vi "Panel.vi"(11 "ImageButtonEditorPanel in":refnum<class "ImageButtonEditorPanel.lvclass">) -> ()   [LabVIEW 2020, in "VolatusGUIControls.lvlib" / "ImageButtonEditorPanel.lvclass"]
uses:
  ImageButtonEditorPanel.lvclass
  C:/dev/lv20CE/relink/volatus-gui-controls/VolatusGUIEditorCore/ElementEditorPanel/ElementEditorPanel.lvclass
  C:/dev/lv20CE/relink/lv-oopanel/OOPanel/Panel/Panel.lvclass
  lv-oopanel/OOPanel/Panel/Basic UI State.ctl
  lv-autocomplete/AutoComplete/AutoComplete/AutoComplete.lvclass/AutoComplete.ctl
  ImageButtonEditorPanel.lvclass/ImageButtonEditorPanel.ctl
  lv-autocomplete/AutoComplete/Launch Autocomplete Handler.vi
  lv-autocomplete/AutoComplete/AutoComplete/AutoComplete.lvclass
  lv-oopanel/OOPanel/Panel/Panel.lvclass
  lv-oopanel/OOPanel/OOPanel.lvlib
  VolatusGUIEditorCore/ElementEditorPanel/ElementEditorPanel.lvclass
  VolatusGUIEditorCore/VolatusGUIEditorCore.lvlib
  lv-web-crypto/lv-base64/Base64.lvlib
  C:/dev/lv20CE/relink/volatus-gui-controls/VolatusGUIControls/ImageButtonEditorPanel/ImageButtonEditorPanel.lvclass
panel:
  out "Last True Image":string
  out "Last False Image":string
  out "Last Image Folder":path
  in  "Top":i32
  in  "Left":i32
  in  "Select True":bool
  in  "Select False":bool
  out "True":picture
  out "False":picture
  in  "Label Text Color":u32(colorbox) caption="Color"
  in  "Label Visible":bool caption="Visible"
  in  "Label":string
  in  "Channel":string
  # "Label"
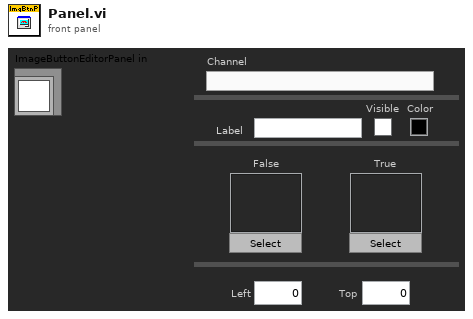
[diagram p1: front panel]
types:
  T1 = typedef "OOPanel.lvlib/Panel.lvclass/Basic UI State.ctl" = enum16{"Init", "Run", "Close"}
  T2 = typedef "VolatusGUIEditorCore.lvlib/ElementEditorPanel.lvclass/Incoming Events.ctl" = cluster{"Update Control":refnum<user-event>}
  T3 = typedef "OOPanel.lvlib/Panel.lvclass/Panel Events.ctl" = cluster{"Visbility":refnum<user-event>, "Close":refnum<user-event>}
  T4 = typedef "VolatusGUIControls.lvlib/ImageButtonEditorPanel.lvclass/Props.ctl" = cluster{"JSON":T5, "Label":T6, "Position":T7}
  T5 = typedef "VolatusGUIControls.lvlib/ImageButtonEditorPanel.lvclass/JSON Props.ctl" = cluster{"Channel":string, "FalseImage":string, "TrueImage":string}
  T6 = typedef "VolatusGUIEditorCore.lvlib/Label Props.ctl" = cluster{"Text":string, "Text Color":u32, "Visible":bool}
  T7 = typedef "VolatusGUIEditorCore.lvlib/Position Props.ctl" = cluster{"Left":i32, "Top":i32}
  T8 = typedef "OOPanel.lvlib/Visibility State.ctl" = enum16{"Idle", "Closed", "Hidden", "Visible", "Subpanel", "Hidden Subpanel"}
  T9 = cluster{"Label":string, "Label Text Color":u32, "Label Visible":bool}
  T10 = typedef "imagedata.ctl" = cluster{"image type":i32, "image depth":i32, "image":u8[], "mask":u8[], "colors":u32[], "Rectangle":cluster{"left":i16, "top":i16, "right":i16, "bottom":i16}}
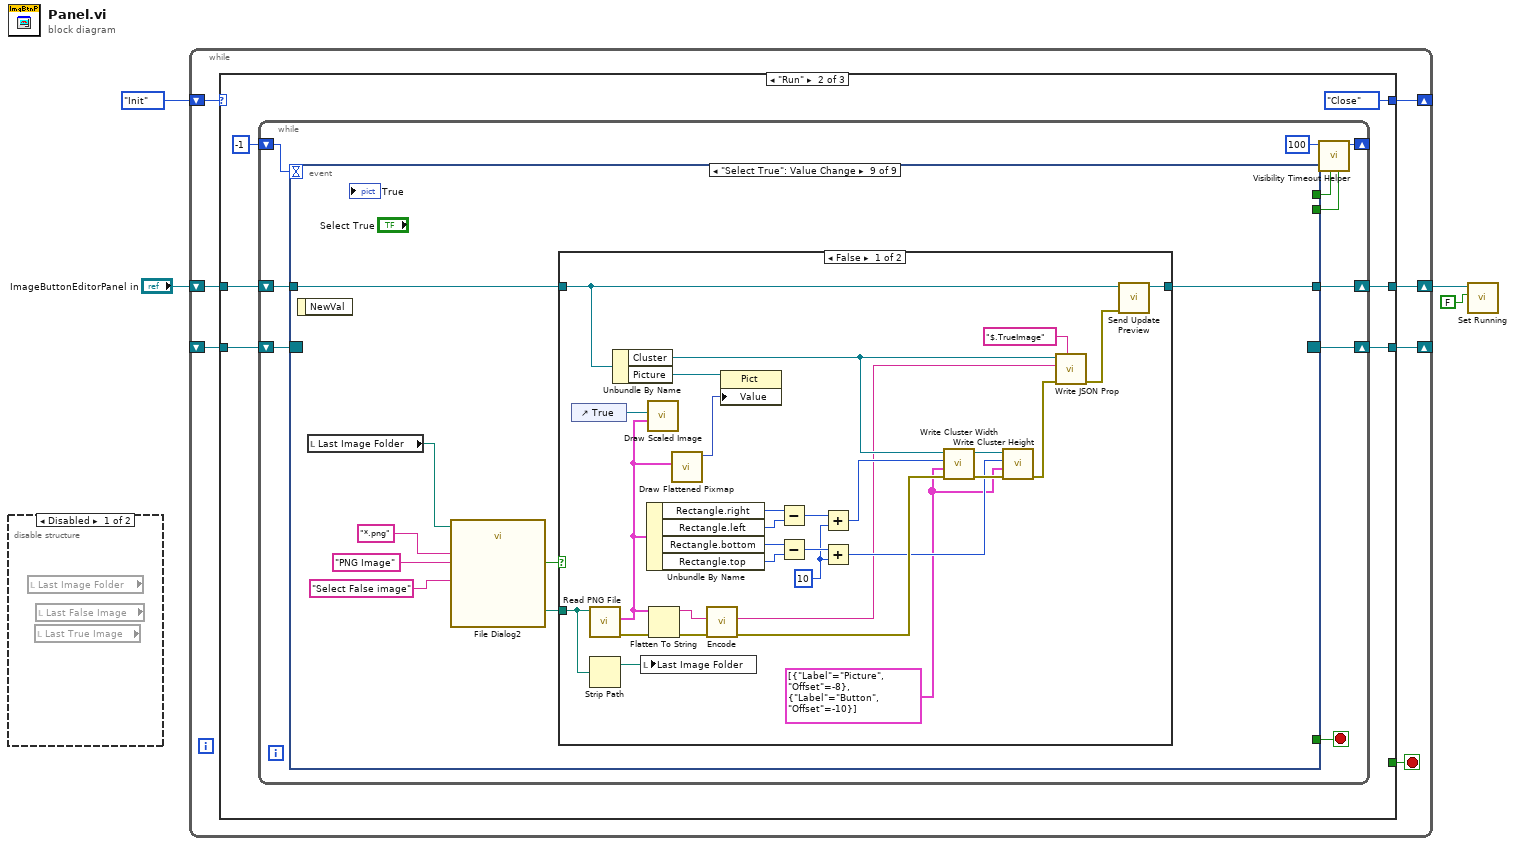
[diagram p0: block diagram]
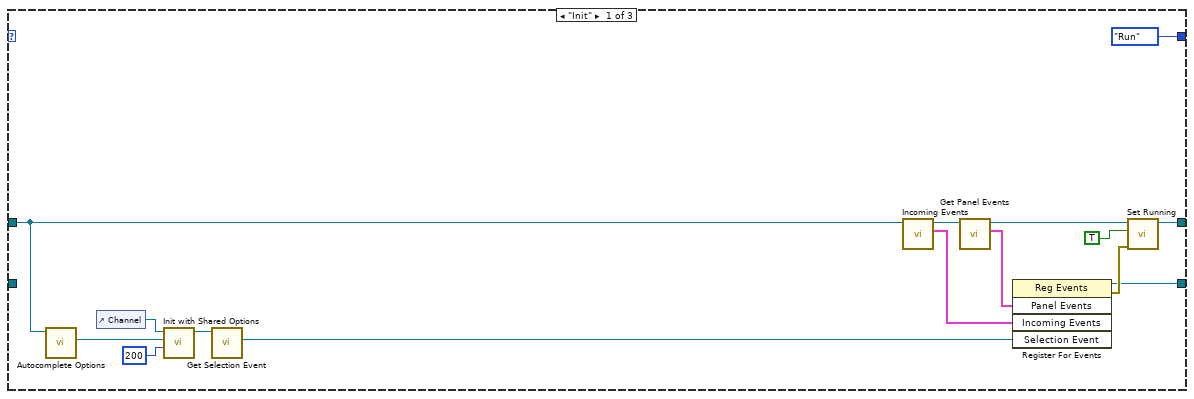
[diagram p3: hidden frame]
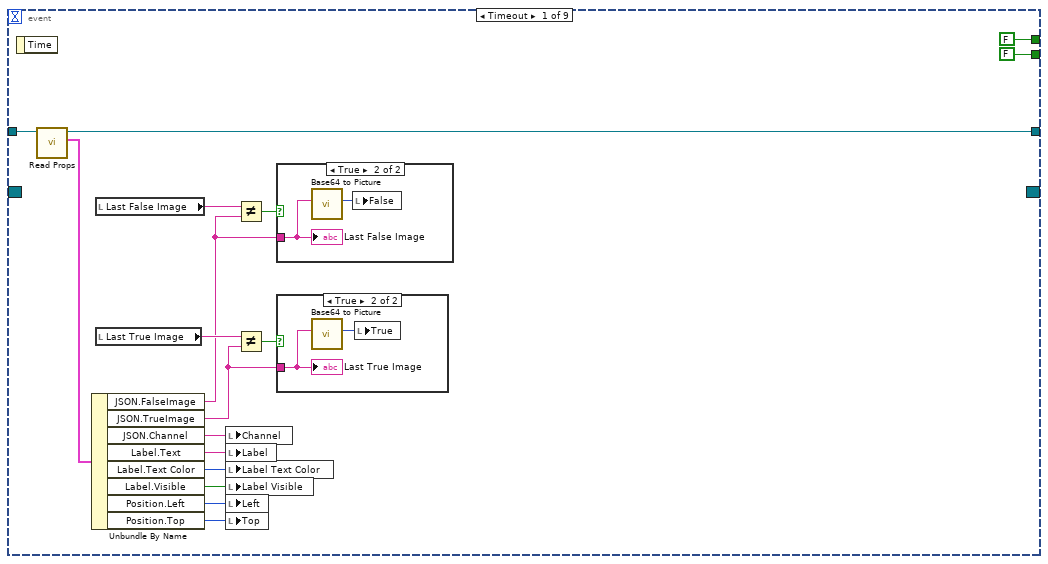
[diagram p4: hidden frame]
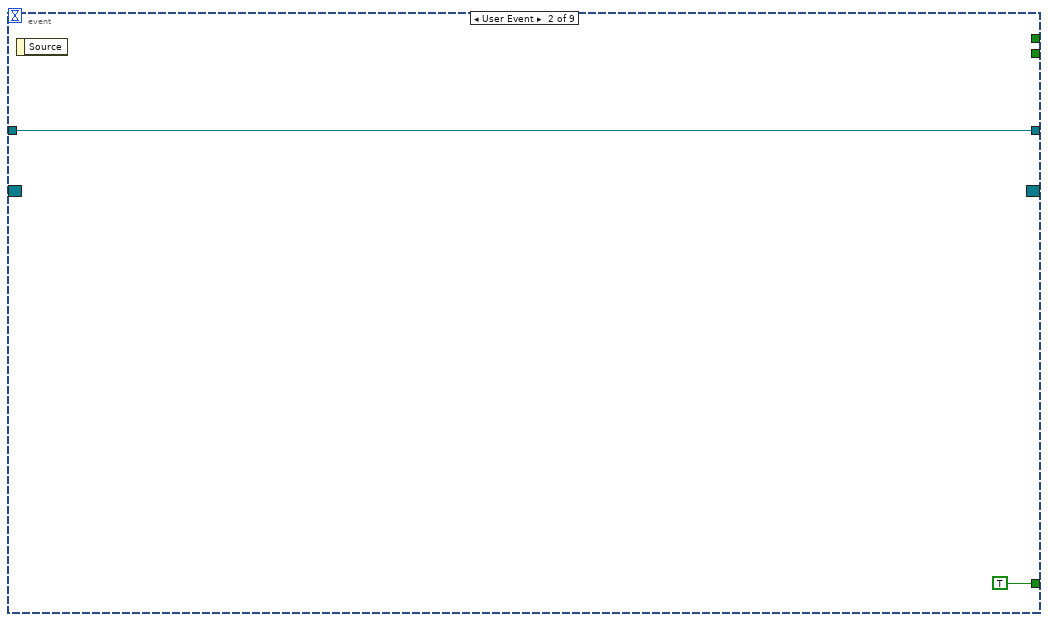
[diagram p7: hidden frame]
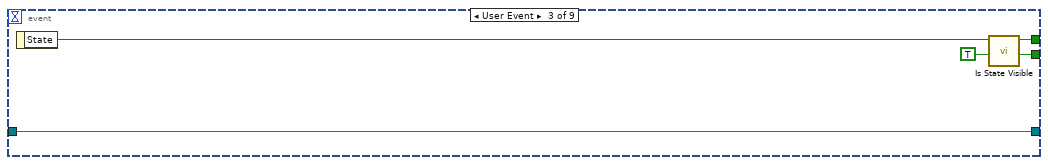
[diagram p8: hidden frame]
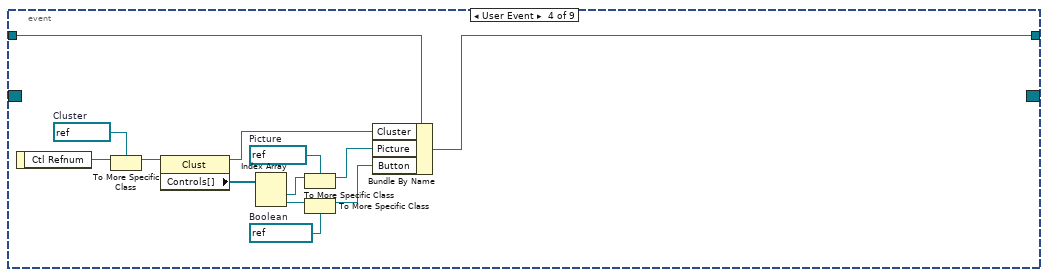
[diagram p9: hidden frame]
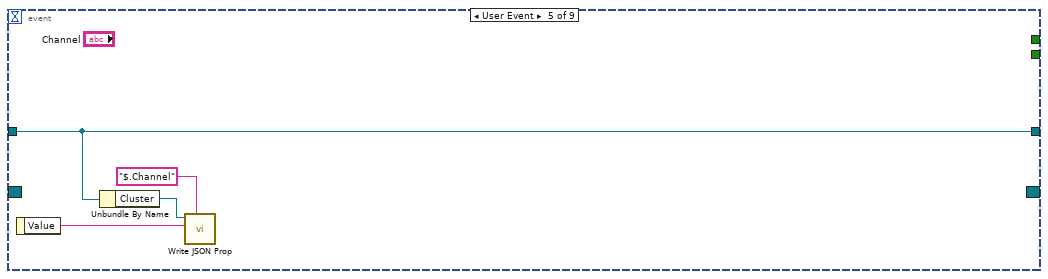
[diagram p10: hidden frame]
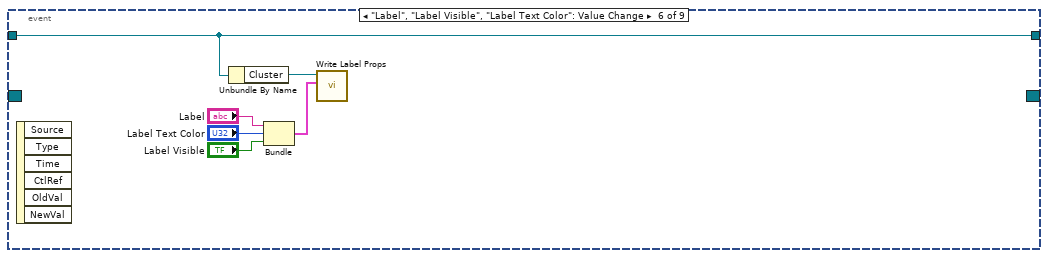
[diagram p11: hidden frame]
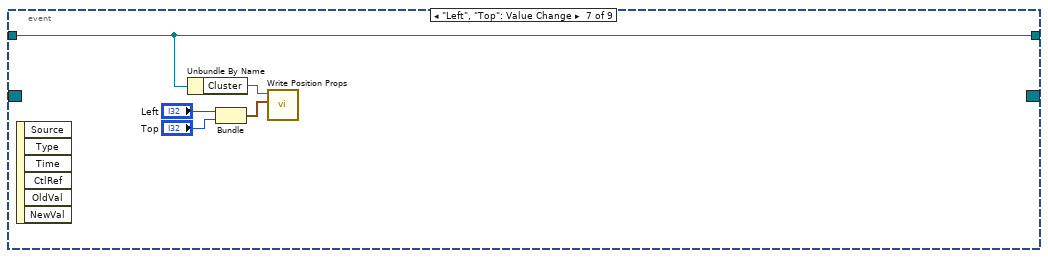
[diagram p12: hidden frame]
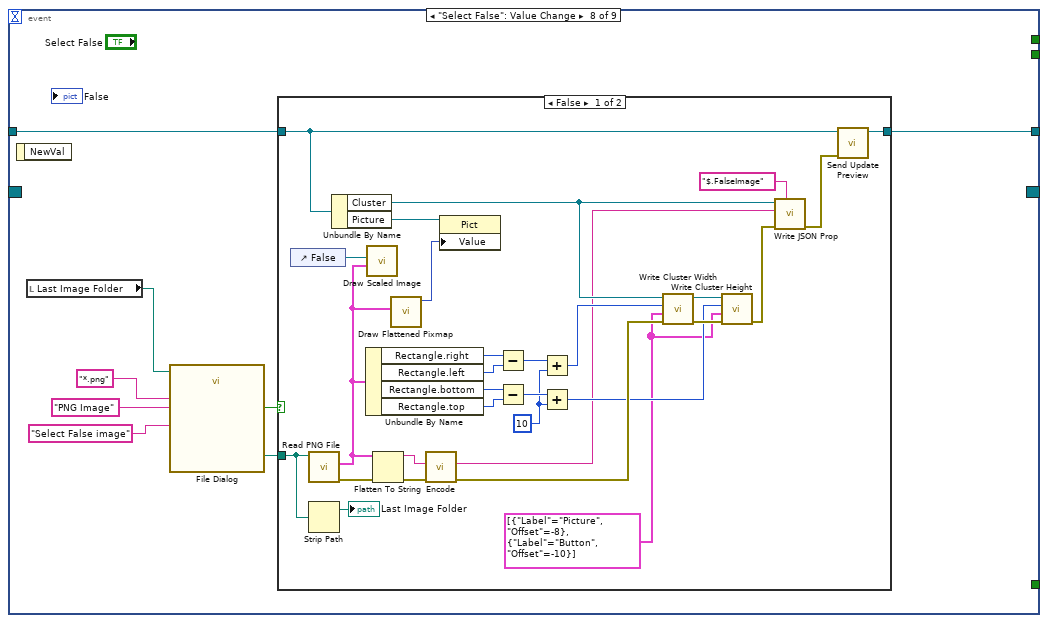
[diagram p13: hidden frame]
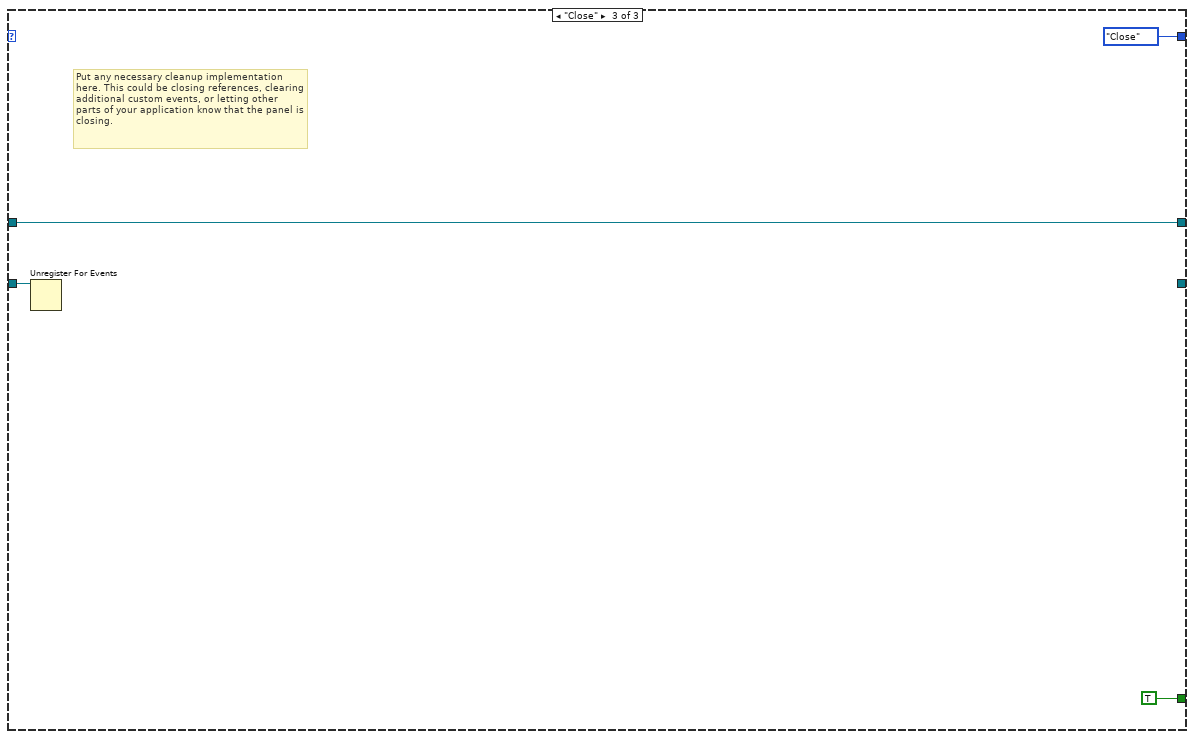
[diagram p16: hidden frame]
diagram:
  n1 = disable-structure shown="Disabled" {
    frame Disabled {
      n2 = local read "Last Image Folder"() -> ()  [unwired: 1 out]
      n3 = local read "Last True Image"() -> ()  [unwired: 1 out]
      n4 = local read "Last False Image"() -> ()  [unwired: 1 out]
    }
    frame Enabled {
    }
  }
  n5 = while {
    shift-right: [w10] -> _
    shift-left: _ -> [w11]
    shift-right: [w8] -> _
    shift-left: Basic_UI_State."Init" ("Basic UI State") -> [w9]
    shift-right: [w6] -> w4
    shift-left: "ImageButtonEditorPanel in" -> [w5]
    stop <- w7 stop-if-true
    n6 = case shown="\"Run\"" w9 {
      tunnel: w11 -> [_ w32 w175]
      tunnel: [w23 w30 _] -> w10
      tunnel: [Basic_UI_State."Run" ("Basic UI State") Basic_UI_State."Close" ("Basic UI State") Basic_UI_State."Close" ("Basic UI State")] -> w8
      tunnel: [_ _ TRUE] -> w7
      tunnel: [w22 w27 w174] -> w6
      tunnel: w5 -> [w14 w28 w174]
      frame "Init" {
        n7 = call "Autocomplete Options.vi"("ElementEditorPanel in"=w14) -> ("Autocomplete Options"=w17:refnum<class "Shared Options.lvclass">)  [unwired: 10 in]
        n8 = control-ref of="Channel"() -> (w13:refnum<vi>)
        n9 = call "Init with Shared Options.vi"("Height (200)"=i16 200, "Shared Options"=w17, "Str Refnum"=w13) -> ("AutoComplete out"=w16:refnum<class "AutoComplete.lvclass">)  [unwired: 7 in, 1 out]
        n10 = call "Get Selection Event.vi"("AutoComplete in"=w16) -> ("Selection Event"=w12:refnum<user-event>)  [unwired: 9 in, 1 out]
        n11 = call "Incoming Events.vi"("ElementEditorPanel in"=w14) -> ("Incoming Events"=w18:T2, "ElementEditorPanel out"=w19:refnum<class "ImageButtonEditorPanel.lvclass">)  [unwired: 9 in]
        n12 = call "Get Panel Events.vi"("Panel in"=w19) -> ("Panel Events"=w20:T3, "Panel out"=w21:refnum<class "ImageButtonEditorPanel.lvclass">)  [unwired: 8 in, 1 out]
        n13 = register-events(w20, w18, w12) -> (reference out=w23:refnum<event-registration>, error out=w25:errorcluster)  [unwired: 2 in]
        n14 = call "Set Running.vi"("error in (no error)"=w25, "Running"=TRUE, "Panel in"=w21) -> ("Panel out"=w22:refnum<class "ImageButtonEditorPanel.lvclass">)  [unwired: 7 in, 1 out]
      }
      frame "Run" {
        n15 = while {
          shift-right: [w38] -> w30
          shift-left: w32 -> [w39]
          shift-right: [w41] -> _
          shift-left: -1 ("Timeout") -> [w40]
          shift-right: [w33] -> w27
          shift-left: w28 -> [w34]
          stop <- w35 stop-if-true
          n16 = event shown="[8] \"Select True\": Value Change" {
            selector: w39 -> [_ _ _ _ _ _ _ _ _]
            dyn-events: [_ _ _ _ _ _ _ _ _] -> w38
            timeout: w40 -> [_ _ _ _ _ _ _ _ _]
            tunnel: [FALSE _ w68 _ _ _ _ _ _] -> w37
            tunnel: [FALSE _ TRUE _ _ _ _ _ _] -> w36
            tunnel: [_ TRUE _ _ _ _ _ _ _] -> w35
            tunnel: w34 -> [w55 w64 w66 w82 w84 w88 w94 w100 w138]
            tunnel: [w56 w64 w66 w73 w84 w88 w94 w99 w137] -> w33
            event Timeout {
              n17 = event-data() -> ()  [unwired: 1 in, 1 out]
              n18 = call "Read Props.vi"("ImageButtonEditorPanel in"=w55) -> ("Props"=w57:T4, "ImageButtonEditorPanel out"=w56:refnum<class "ImageButtonEditorPanel.lvclass">)  [unwired: 8 in, 1 out]
              n19 = Unbundle By Name(w57) -> ("JSON.FalseImage"=w45:string, "JSON.TrueImage"=w43:string, "JSON.Channel"=w54:string, "Label.Text"=w52:string, "Label.Text Color"=w51:u32, "Label.Visible"=w50:bool, "Position.Left"=w49:i32, "Position.Top"=w53:i32)
              n20 = local read "Last False Image"() -> (w48:string)
              n21 = local read "Last True Image"() -> (w47:string)
              n22 = local write "Channel"(w54) -> ()
              n23 = local write "Label"(w52) -> ()
              n24 = local write "Label Text Color"(w51) -> ()
              n25 = local write "Label Visible"(w50) -> ()
              n26 = local write "Left"(w49) -> ()
              n27 = local write "Top"(w53) -> ()
              n28 = Not Equal?(x=w48, y=w45) -> (x != y?=w46:bool)
              n29 = Not Equal?(x=w47, y=w43) -> (x != y?=w44:bool)
              n30 = case shown="True" w46 {
                tunnel: w45 -> [_ w63]
                frame False {
                }
                frame True {
                  n31 = call "Base64 to Picture.vi"("Base64 PNG Data"=w63) -> ("Picture"=w62:picture)  [unwired: 9 in, 1 out]
                  n32 = local write "False"(w62) -> ()
                  "Last False Image" <- w63
                }
              }
              n33 = case shown="True" w44 {
                tunnel: w43 -> [_ w61]
                frame False {
                }
                frame True {
                  n34 = call "Base64 to Picture.vi"("Base64 PNG Data"=w61) -> ("Picture"=w60:picture)  [unwired: 9 in, 1 out]
                  n35 = local write "True"(w60) -> ()
                  "Last True Image" <- w61
                }
              }
            }
            event User Event {
              n36 = event-data() -> ()  [unwired: 1 in, 1 out]
            }
            event User Event {
              n37 = event-data() -> ("State"=w69:T8)  [unwired: 1 in]
              n38 = call "Is State Visible.vi"("Visibility"=w69) -> ("Visible"=w68:bool)  [unwired: 10 in]
            }
            event User Event {
              w75 = refnum<vi> refnum  # Boolean
              w77 = refnum<vi> refnum  # Picture
              w80 = refnum<vi> refnum  # Cluster
              n39 = event-data() -> ("Ctl Refnum"=w81:refnum<vi>)  [unwired: 1 in]
              n40 = To More Specific Class(target class=w80, reference=w81) -> (specific class reference=w79:refnum<vi>)  [unwired: 1 in, 1 out]
              n41 = property class="Clust"(reference=w79) -> (reference out=w72:refnum<vi>, "Controls[]"=w78:refnum<vi>[])  [unwired: 1 in, 1 out]
              n42 = Index Array(array=w78) -> (element #1=w76:refnum<vi>, element #2=w74:refnum<vi>)  [unwired: 2 in]
              n43 = To More Specific Class(target class=w77, reference=w76) -> (specific class reference=w71:refnum<vi>)  [unwired: 1 in, 1 out]
              n44 = To More Specific Class(target class=w75, reference=w74) -> (specific class reference=w70:refnum<vi>)  [unwired: 1 in, 1 out]
              n45 = Bundle By Name(cluster=w82, "Cluster"=w72, "Picture"=w71, "Button"=w70) -> (w73:refnum<class "ImageButtonEditorPanel.lvclass">)
            }
            event User Event {
              n46 = event-data() -> ("Value"=w83:string)  [unwired: 1 in]
              n47 = Unbundle By Name(w84) -> ("Cluster"=w86:refnum<vi>)
              n48 = call "Write JSON Prop.vi"("JSON Path"="$.Channel" ("$Path or Item Name"), "Value"=w83, "Ctl Refnum in"=w86) -> ()  [unwired: 7 in, 2 out]
            }
            event "Label", "Label Visible", "Label Text Color": Value Change {
              n49 = event-data() -> ()  [unwired: 1 in, 6 out]
              n50 = Unbundle By Name(w88) -> ("Cluster"=w87:refnum<vi>)
              n51 = Bundle("Label"="Label", "Label Text Color"="Label Text Color", "Label Visible"="Label Visible") -> (w89:T9)  [unwired: 1 in]
              n52 = call "Write Label Props.vi"("Label Props"=w89, "Ctl Refnum in"=w87) -> ()  [unwired: 8 in, 2 out]
            }
            event "Left", "Top": Value Change {
              n53 = event-data() -> ()  [unwired: 1 in, 6 out]
              n54 = Unbundle By Name(w94) -> ("Cluster"=w93:refnum<vi>)
              n55 = Bundle("Left"="Left", "Top"="Top") -> (w95:cluster{"Left":i32, "Top":i32})  [unwired: 1 in]
              n56 = call "Write Position Props.vi"("Position Props"=w95, "Ctl Refnum in"=w93) -> ()  [unwired: 8 in, 2 out]
            }
            event "Select False": Value Change {
              n57 = event-data() -> ()  [unwired: 1 in, 1 out]
              n58 = local read "Last Image Folder"() -> (w98:path)
              n59 = call "File Dialog"("start path"=w98, "prompt"="Select False image", "pattern (all files)"="*.png", "pattern label"="PNG Image") -> ("selected path"=w101:path, "cancelled"=w102:bool)  [unwired: 8 in, 2 out]
              n60 = case shown="False" w102 {
                tunnel: w101 -> [w131 _]
                tunnel: w100 -> [w115 w135]
                tunnel: [w114 w135] -> w99
                frame False {
                  w120 = cluster{"Label":string, "Offset":i32}[] [{"Label"="Picture", "Offset"=-8}, {"Label"="Button", "Offset"=-10}] ("Nested Offsets (None)")
                  w124 = i16 10 ("y")
                  n61 = control-ref of="False"() -> (w112:refnum<vi>)
                  n62 = call <vilib>:"Read PNG File.vi"("path to PNG file"=w131) -> ("error out"=w109:errorcluster, "image data"=w106:T10)  [unwired: 8 in, 1 out]
                  n63 = Strip Path(path=w131) -> (stripped path=→"Last Image Folder":path)  [unwired: 1 out]
                  n64 = Unbundle By Name(w115) -> ("Cluster"=w119:refnum<vi>, "Picture"=w111:refnum<vi>)
                  n65 = Unbundle By Name(w106) -> ("Rectangle.right"=w130:i16, "Rectangle.left"=w129:i16, "Rectangle.bottom"=w128:i16, "Rectangle.top"=w127:i16)
                  n66 = call "Draw Scaled Image.vi"("Image"=w106, "Picture Ref"=w112) -> ()  [unwired: 10 in]
                  n67 = Flatten To String(anything=w106, error in (no error)=w109) -> (data string=w107:string, error out=w108:errorcluster)  [unwired: 2 in, 1 out]
                  n68 = call <vilib>:"Draw Flattened Pixmap.vi"("image data"=w106) -> ("new picture"=w110:picture)  [unwired: 8 in]
                  n69 = call "Encode.vi"("error in (no error)"=w108, "string in (not encoded)"=w107) -> ("error out"=w134:errorcluster, "string out (base64-encoded)"=w117:string)  [unwired: 8 in]
                  n70 = property class="Pict"(reference=w111, "Value"=w110) -> ()  [unwired: 1 in, 2 out]
                  n71 = Subtract(x=w130, y=w129) -> (x-y=w126:i16)
                  n72 = Subtract(x=w128, y=w127) -> (x-y=w125:i16)
                  n73 = Add(x=w126, y=w124) -> (x+y=w123:i16)
                  n74 = Add(x=w125, y=w124) -> (x+y=w121:i16)
                  n75 = call "Write Cluster Width.vi"("error in (no error)"=w134, "Nested Offsets (None)"=w120, "Width"=w123, "Cluster in"=w119) -> ("error out"=w133:errorcluster, "Cluster"=w122:refnum<vi>)  [unwired: 6 in]
                  n76 = call "Write Cluster Height.vi"("error in (no error)"=w133, "Nested Offsets (None)"=w120, "Height"=w121, "Cluster in"=w122) -> ("error out"=w116:errorcluster)  [unwired: 6 in, 1 out]
                  n77 = call "Write JSON Prop.vi"("JSON Path"="$.FalseImage", "error in (no error)"=w116, "Value"=w117, "Ctl Refnum in"=w119) -> ("error out"=w113:errorcluster)  [unwired: 6 in, 1 out]
                  n78 = call "Send Update Preview.vi"("error in (no error)"=w113, "ElementEditorPanel in"=w115) -> ("ElementEditorPanel out"=w114:refnum<class "ImageButtonEditorPanel.lvclass">)  [unwired: 8 in, 1 out]
                }
                frame True {
                }
              }
            }
            event "Select True": Value Change {
              n79 = event-data() -> ()  [unwired: 1 in, 1 out]
              n80 = local read "Last Image Folder"() -> (w136:path)
              n81 = call "File Dialog2"("start path"=w136, "prompt"="Select False image", "pattern (all files)"="*.png", "pattern label"="PNG Image") -> ("selected path"=w139:path, "cancelled"=w140:bool)  [unwired: 8 in, 2 out]
              n82 = case shown="False" w140 {
                tunnel: w139 -> [w170 _]
                tunnel: w138 -> [w151 w173]
                tunnel: [w150 w173] -> w137
                frame False {
                  w158 = cluster{"Label":string, "Offset":i32}[] [{"Label"="Picture", "Offset"=-8}, {"Label"="Button", "Offset"=-10}] ("Nested Offsets (None)")
                  w162 = i16 10 ("y")
                  n83 = control-ref of="True"() -> (w145:refnum<vi>)
                  n84 = call <vilib>:"Read PNG File.vi"("path to PNG file"=w170) -> ("error out"=w155:errorcluster, "image data"=w147:T10)  [unwired: 8 in, 1 out]
                  n85 = Strip Path(path=w170) -> (stripped path=w144:path)  [unwired: 1 out]
                  n86 = Unbundle By Name(w151) -> ("Cluster"=w157:refnum<vi>, "Picture"=w148:refnum<vi>)
                  n87 = local write "Last Image Folder"(w144) -> ()
                  n88 = Unbundle By Name(w147) -> ("Rectangle.right"=w168:i16, "Rectangle.left"=w167:i16, "Rectangle.bottom"=w166:i16, "Rectangle.top"=w165:i16)
                  n89 = call "Draw Scaled Image.vi"("Image"=w147, "Picture Ref"=w145) -> ()  [unwired: 10 in]
                  n90 = Flatten To String(anything=w147, error in (no error)=w155) -> (data string=w169:string, error out=w154:errorcluster)  [unwired: 2 in, 1 out]
                  n91 = call <vilib>:"Draw Flattened Pixmap.vi"("image data"=w147) -> ("new picture"=w146:picture)  [unwired: 8 in]
                  n92 = call "Encode.vi"("error in (no error)"=w154, "string in (not encoded)"=w169) -> ("error out"=w172:errorcluster, "string out (base64-encoded)"=w153:string)  [unwired: 8 in]
                  n93 = property class="Pict"(reference=w148, "Value"=w146) -> ()  [unwired: 1 in, 2 out]
                  n94 = Subtract(x=w168, y=w167) -> (x-y=w164:i16)
                  n95 = Subtract(x=w166, y=w165) -> (x-y=w163:i16)
                  n96 = Add(x=w164, y=w162) -> (x+y=w161:i16)
                  n97 = Add(x=w163, y=w162) -> (x+y=w159:i16)
                  n98 = call "Write Cluster Width.vi"("error in (no error)"=w172, "Nested Offsets (None)"=w158, "Width"=w161, "Cluster in"=w157) -> ("error out"=w171:errorcluster, "Cluster"=w160:refnum<vi>)  [unwired: 6 in]
                  n99 = call "Write Cluster Height.vi"("error in (no error)"=w171, "Nested Offsets (None)"=w158, "Height"=w159, "Cluster in"=w160) -> ("error out"=w152:errorcluster)  [unwired: 6 in, 1 out]
                  n100 = call "Write JSON Prop.vi"("JSON Path"="$.TrueImage", "error in (no error)"=w152, "Value"=w153, "Ctl Refnum in"=w157) -> ("error out"=w149:errorcluster)  [unwired: 6 in, 1 out]
                  n101 = call "Send Update Preview.vi"("error in (no error)"=w149, "ElementEditorPanel in"=w151) -> ("ElementEditorPanel out"=w150:refnum<class "ImageButtonEditorPanel.lvclass">)  [unwired: 8 in, 1 out]
                }
                frame True {
                }
              }
            }
          }
          n102 = call "Visibility Timeout Helper.vi"("Update?"=w36, "Use Timeout?"=w37, "Visible Timeout mS"=100) -> ("Timeout"=w41:i32)  [unwired: 8 in]
        }
      }
      frame "Close" {
        # "Put any necessary cleanup implementation here. This could be closing references, clearing additional custom events, or letting other parts of your application know that the panel is closing."
        n103 = Unregister For Events(event registration refnum=w175) -> ()  [unwired: 1 in, 1 out]
      }
    }
  }
  n104 = call "Set Running.vi"("Running"=FALSE, "Panel in"=w4) -> ()  [unwired: 8 in, 2 out]
